vi "YW_ziExample-PollDemod.vi"(0 "Address":string="DEV", 1 "stop":bool) -> (20 "Selected Device":string)   [LabVIEW 2016]
doc: "Control a Zurich instrument device via the LabOne Labview API. \nRequirements: Zurich Instruments MFLI, HF2 or UHFLI \nThis example polls demod data for a given time from the instrument.\n\n© Zurich Instruments AG, www.zhinst.com"
uses:
  <instrlib>/Zurich Instruments LabOne/Public/Utility/ziTicksToS_vector.vi
  <instrlib>/Zurich Instruments LabOne/Zurich Instruments LabOne.lvlib
panel:
  out "size(s)":i32
  out "Timestamps (ticks)":u64[](array[numeric])
  out "Waveform Chart":dbl[](graph)
  in  "Subscribe Path Array":string[](array[string])=["demods/0/sample"]
  out "Error Out":errorcluster
  out "XY Graph":cluster{dbl[], "X (Vrms)":dbl[]}[](graph)
  in  "time":dbl=1.0 caption="recording time [s]"
  # "ziExample-PollDemod.vi\nRequirements: HF2, UHFLI or MFLI\nsee block diagram for VI description"
  # "Tested Instruments:\n- MFLI\n- HF2LI\n- UHFLI"
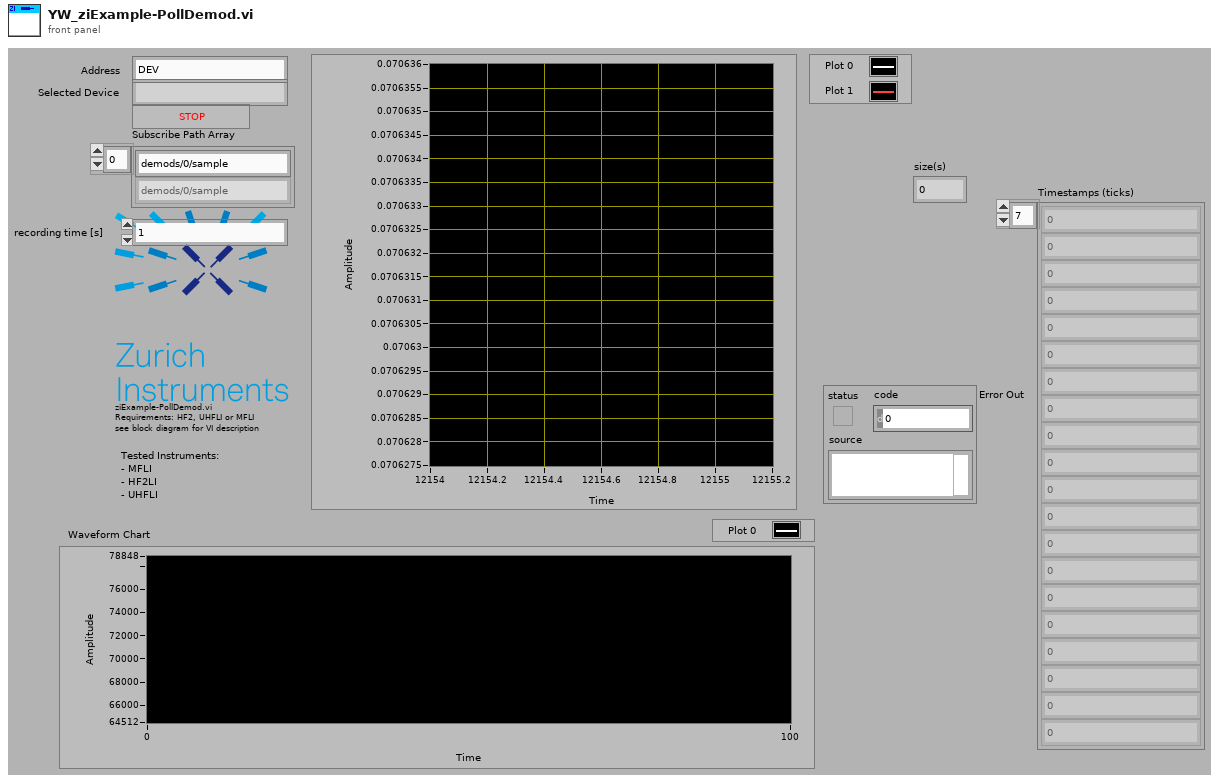
[diagram p1: front panel]
types:
  T1 = typedef "Zurich Instruments LabOne.lvlib/ziTypeHandle.ctl" = cluster{"handleValid":bool, "Conn":u64, "Path Prefix":string, "Handle":u64, "Connected":bool, "Clockbase(s)":dbl}
  T2 = typedef "Zurich Instruments LabOne.lvlib/ziTypeDemodSampleEx.ctl" = cluster{"Timestamps (ticks)":u64[], "X (Vrms)":dbl[], "Y (Vrms)":dbl[], "Osc Phase (rad)":dbl[], "Freq (Hz)":dbl[], "DIO":u32[], "Aux In 0 (V)":dbl[], "Aux In 1 (V)":dbl[], "Trigger":u32[]}
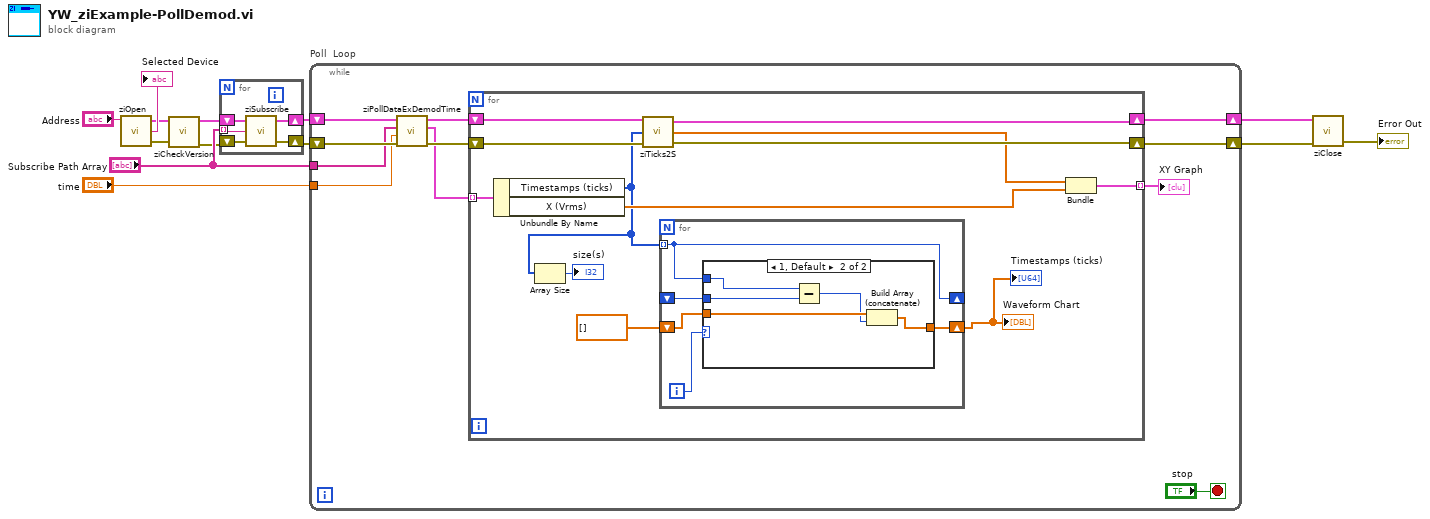
[diagram p0: block diagram]
diagram:
  n1 = call <instrlib>:"ziOpen.vi"("Address"="Address") -> ("Error Out"=w3:errorcluster, "Selected Device"=→"Selected Device":string, "HandleOut"=w4:T1)  [unwired: 1 in, 2 out]
  n2 = call <instrlib>:"ziCheckVersion.vi"("Handle In"=w4, "Error In"=w3) -> ("Handle Out"=w1:T1, "Error Out"=w2:errorcluster)  [unwired: 12 in]
  n3 = for {
    tunnel: "Subscribe Path Array" -> [w14] mode=indexing
    shift-right: [w16] -> w9
    shift-left: w2 -> [w17]
    shift-right: [w15] -> w8
    shift-left: w1 -> [w18]
    n4 = call <instrlib>:"ziSubscribe.vi"("error in"=w17, "Path ()"=w14, "Handle In"=w18) -> ("error out"=w16:errorcluster, "Handle Out"=w15:T1)  [unwired: 1 in]
  }
  n5 = while "Poll  Loop" {
    shift-right: [w23] -> w13
    shift-left: w8 -> [w27]
    shift-right: [w22] -> w10
    shift-left: w9 -> [w28]
    tunnel: "Subscribe Path Array" -> [w26]
    tunnel: "time" -> [w21]
    stop <- "stop" stop-if-true
    n6 = call <instrlib>:"ziPollDataExDemodTime.vi"("error in"=w28, "recording time (1) [s]"=w21, "SubscribepathArray"=w26, "Handle In"=w27) -> ("error out"=w25:errorcluster, "Demod Sample Out"=w19:T2[], "Handle Out"=w24:T1)  [unwired: 5 in]
    n7 = for {
      tunnel: w19 -> [w37] mode=indexing
      shift-right: [w38] -> w22
      shift-left: w25 -> [w41]
      shift-right: [w39] -> w23
      shift-left: w24 -> [w40]
      tunnel: [w36] -> w20 mode=indexing
      n8 = Unbundle By Name(w37) -> ("Timestamps (ticks)"=w30:u64[], "X (Vrms)"=w35:dbl[])
      n9 = Array Size(array=w30) -> (size(s)=→"size(s)":i32)
      n10 = call-poly <instrlib>:"ziTicks2S.vi"("Error In"=w41, "Timestamp (ticks)"=w30, "Handle In"=w40) -> ("Error Out"=w38:errorcluster, "Timestamp(s)"=w33:dbl[], "Handle Out"=w39:T1)
      n11 = for {
        tunnel: w30 -> [w46] mode=indexing
        shift-right: [w46] -> _
        shift-left: _ -> [w45]
        shift-right: [w42] -> w32
        shift-left: dbl[] [] -> [w43]
        i -> [w44]
        n12 = case shown="1, Default" w44 {
          tunnel: w46 -> [_ w52]
          tunnel: w45 -> [_ w51]
          tunnel: w43 -> [w47 w50]
          tunnel: [w47 w48] -> w42
          frame 0 {
          }
          frame 1, Default {
            n13 = Subtract(x=w52, y=w51) -> (x-y=w49:u64)
            n14 = Build Array (concatenate)(w50, w49) -> (w48:dbl[])
          }
        }
      }
      "Waveform Chart" <- w32
      "Timestamps (ticks)" <- w32
      n15 = Bundle("Timestamp(s)"=w33, "X (Vrms)"=w35) -> (w36:cluster{"Timestamp(s)":dbl[], "X (Vrms)":dbl[]})  [unwired: 1 in]
    }
    "XY Graph" <- w20
  }
  n16 = call <instrlib>:"ziClose.vi"("Error In"=w10, "Handle In"=w13) -> ("Error Out"=→"Error Out":errorcluster)  [unwired: 3 out]
